vi "Convert Speed Units to Device Units.vi"(9 "Microstep Size (0)":dbl, 10 "Units (0: device speed units)":u16(ring) items=["device speed units", "microns per second", "millimeters per second", "inches per second", "degrees per second"], 11 "Speed (0)":dbl) -> (1 "Device Speed (64-bit)":i64, 2 "Device Speed (String)":string, 3 "Device Speed (32-bit)":i32)   [LabVIEW 2020, in "Zaber A Series.lvlib"]
doc: "Helper to convert standard units of speed to device-specific speed units.\n\nEnter a Speed quantity and select a unit to convert from. The output will be that speed expressed in native device speed units. \n\nIf you select a unit other than microsteps or microsteps per second, you must also provide the Microstep Size conversion factor from microsteps to micrometers (for linear devices) or degrees (for rotary devices), which can be found in your device manual."
uses:
  Zaber A Series.lvlib
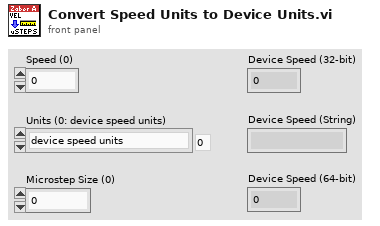
[diagram p1: front panel]
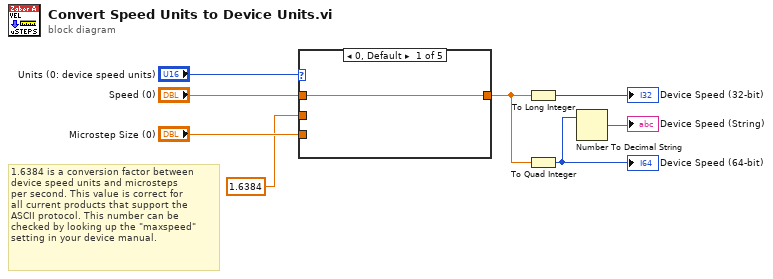
[diagram p0: block diagram]
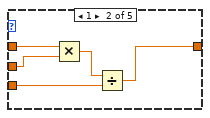
[diagram p2: hidden frame]
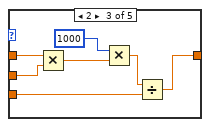
[diagram p3: hidden frame]
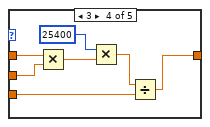
[diagram p4: hidden frame]
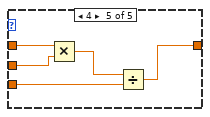
[diagram p5: hidden frame]
diagram:
  # "1.6384 is a conversion factor between \ndevice speed units and microsteps \nper second. This value is correct for\nall current products that support the\nASCII protocol. This number can be \nchecked by looking up the \"maxspeed\"\nsetting in your device manual."
  n1 = case shown="0, Default" "Units (0: device speed units)" {
    tunnel: 1.6384 ("Speed Constant (1.6384)") -> [_ w12 w18 w24 w31]
    tunnel: "Microstep Size (0)" -> [_ w14 w20 w26 w33]
    tunnel: "Speed (0)" -> [w9 w13 w19 w25 w32]
    tunnel: [w9 w10 w15 w22 w29] -> w2
    frame 0, Default {
    }
    frame 1 {
      n2 = Multiply(x=w13, y=w12) -> (x*y=w11:dbl)
      n3 = Divide(x=w11, y=w14) -> (x/y=w10:dbl)
    }
    frame 2 {
      n4 = Multiply(x=w19, y=w18) -> (x*y=w17:dbl)
      n5 = Multiply(x=1000, y=w17) -> (x*y=w21:dbl)
      n6 = Divide(x=w21, y=w20) -> (x/y=w15:dbl)
    }
    frame 3 {
      n7 = Multiply(x=w25, y=w24) -> (x*y=w23:dbl)
      n8 = Multiply(x=25400, y=w23) -> (x*y=w27:dbl)
      n9 = Divide(x=w27, y=w26) -> (x/y=w22:dbl)
    }
    frame 4 {
      n10 = Multiply(x=w32, y=w31) -> (x*y=w30:dbl)
      n11 = Divide(x=w30, y=w33) -> (x/y=w29:dbl)
    }
  }
  n12 = To Long Integer(number=w2) -> (32bit integer=→"Device Speed (32-bit)":i32)
  n13 = To Quad Integer(1:w2) -> (0:w1:i64)
  "Device Speed (64-bit)" <- w1
  n14 = Number To Decimal String(number=w1) -> (decimal integer string=→"Device Speed (String)":string)  [unwired: 1 in]
